vi "FRCts20_WebMethods_Redirect_Notifications.vi"(7 "response code (200)":i32(ring)=200 items=["100"=100, "101"=101, "200"=200, "201"=201, "202"=202, "203"=203, "204"=204, "205"=205, "206"=206, "300"=300, "301"=301, "302"=302, "303"=303, "304"=304, "305"=305, "306"=306, "307"=307, "400"=400, "401"=401, "402"=402, "403"=403, "404"=404, "405"=405, "406"=406, "407"=407, "408"=408, "409"=409, "410"=410, "411"=411, "412"=412, "413"=413, "414"=414, "415"=415, "416"=416, "417"=417, "500"=500, "501"=501, "502"=502, "503"=503, "504"=504, "505"=505], 8 "error in (no error)":errorcluster, 11 "httpRequestID":u32) -> (0 "error out":errorcluster, 3 "httpRequestID out":u32)   [LabVIEW 2013, in "FRCts20_WebMethods.lvlib"]
uses:
  FRCts20_WebMethods.lvlib
  <vilib>/wsapi/NI_WebServices.lvlib
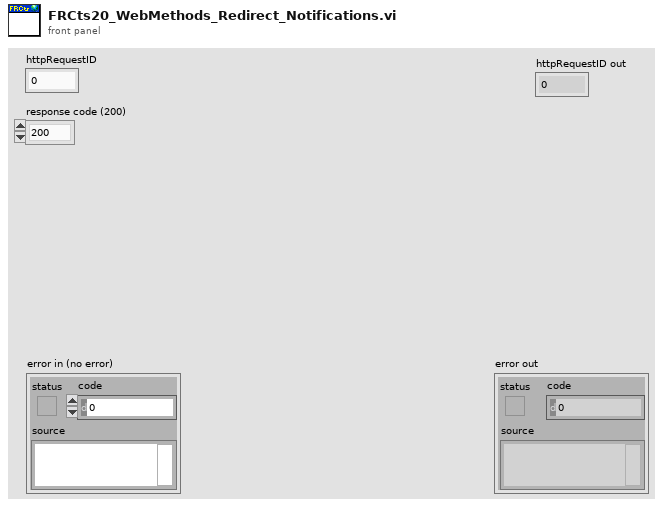
[diagram p1: front panel]
types:
  T1 = typedef "FRCts20_WebMethods.lvlib/FRCts20_WebMethods_ctl_returntype.ctl" = string
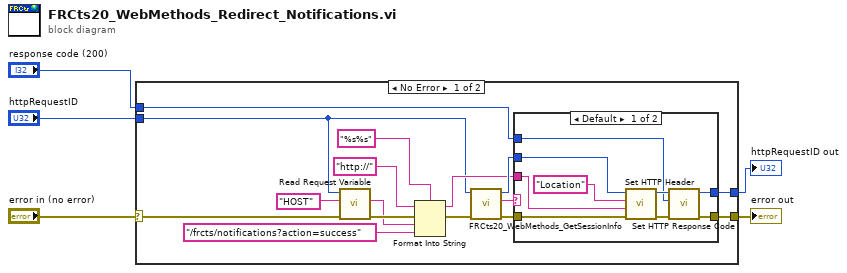
[diagram p0: block diagram]
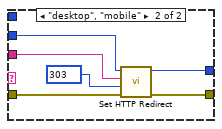
[diagram p2: hidden frame]
diagram:
  n1 = case shown="No Error" "error in (no error)" {
    selector: "error in (no error)" -> [w10 w38]
    tunnel: [w14 w38] -> w5
    tunnel: "httpRequestID" -> [w6 w37]
    tunnel: [w13 w37] -> w3
    tunnel: "response code (200)" -> [w11 _]
    frame No Error {
      n2 = call <vilib>:"Read Request Variable.vi"("error in (no error)"=w10, "variable name"="HOST", "httpRequestID"=w6) -> ("error out"=w9:errorcluster, "value"=w8:string)  [unwired: 6 in, 1 out]
      n3 = Format Into String(format string="%s%s", initial string="http://", error in=w9, w8, "/frcts/notifications?action=success") -> (resulting string=w12:string, error out=w15:errorcluster)
      n4 = call "FRCts20_WebMethods_GetSessionInfo.vi"("error in"=w15, "httpRequestID"=w6) -> ("error out"=w17:errorcluster, "Return Type"=w18:T1, "httpRequestID out"=w16:u32)  [unwired: 7 in]
      n5 = case shown="Default" w18 {
        tunnel: [w26 w36] -> w14
        tunnel: [w23 w35] -> w13
        tunnel: w17 -> [w30 w33]
        tunnel: w16 -> [w29 w32]
        tunnel: w12 -> [w27 w31]
        tunnel: w11 -> [w22 _]
        frame Default {
          n6 = call <vilib>:"Set HTTP Header.vi"("error in (no error)"=w30, "header value"=w27, "header"="Location", "httpRequestID"=w29) -> ("error out"=w25:errorcluster, "httpRequestID out"=w24:u32)  [unwired: 6 in]
          n7 = call <vilib>:"Set HTTP Response Code.vi"("error in (no error)"=w25, "response code (200)"=w22, "httpRequestID"=w24) -> ("error out"=w26:errorcluster, "httpRequestID out"=w23:u32)  [unwired: 7 in]
        }
        frame "desktop", "mobile" {
          w34 = 303 items=["100"=100, "101"=101, "200"=200, "201"=201, "202"=202, "203"=203, "204"=204, "205"=205, "206"=206, "300"=300, "301"=301, "302"=302, "303"=303, "304"=304, "305"=305, "306"=306, "307"=307, "400"=400, "401"=401, "402"=402, "403"=403, "404"=404, "405"=405, "406"=406, "407"=407, "408"=408, "409"=409, "410"=410, "411"=411, "412"=412, "413"=413, "414"=414, "415"=415, "416"=416, "417"=417, "500"=500, "501"=501, "502"=502, "503"=503, "504"=504, "505"=505] ("response code (307)")
          n8 = call <vilib>:"Set HTTP Redirect.vi"("error in (no error)"=w33, "response code (307)"=w34, "redirect URL"=w31, "httpRequestID"=w32) -> ("error out"=w36:errorcluster, "httpRequestID out"=w35:u32)  [unwired: 6 in]
        }
      }
    }
    frame Error {
    }
  }
  "error out" <- w5
  "httpRequestID out" <- w3
